vi "getCardSlot.vi"(1 "Card Index":u16, 2 "initialized array":u16[](array[numeric])) -> (0 "Slot":u16)   [LabVIEW 2011]
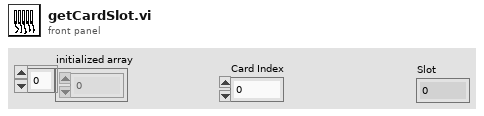
[diagram p1: front panel]
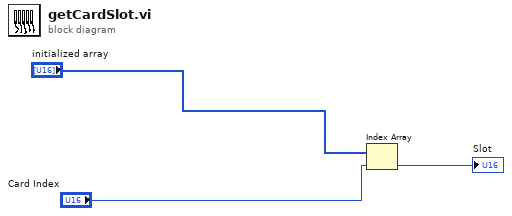
[diagram p0: block diagram]
diagram:
  n1 = Index Array(array="initialized array", index="Card Index") -> (element=→"Slot":u16)
